vi "quickStack.vi"(2 "stackFname":path=path "C:/Users/sims01/Desktop/dataAcq/data.dcimg", 3 "noFrames":i32, 4 "sCMOShandle":u32, 5 "imgAcqDelay":u32) -> (0 "stackComplete":bool, 1 "timeTaken":u32)   [LabVIEW 2015]
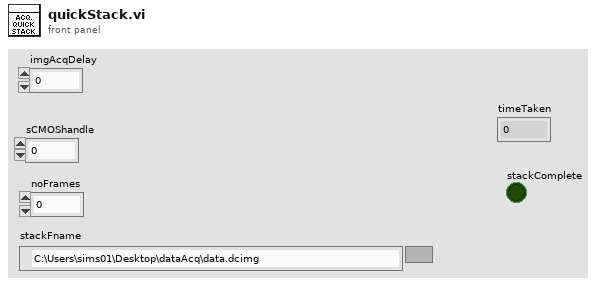
[diagram p1: front panel]
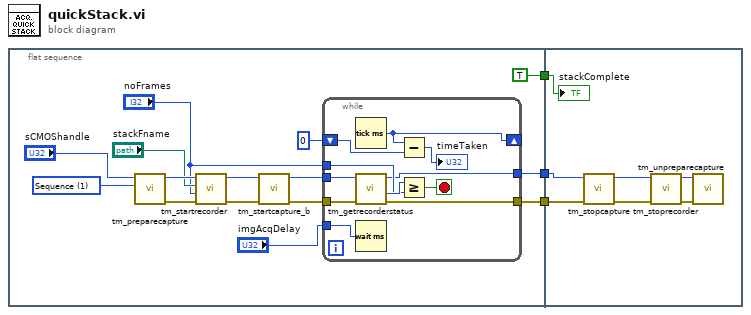
[diagram p0: block diagram]
diagram:
  n1 = flat-sequence {
    tunnel: [TRUE] -> w3
    tunnel: [w5] -> w2
    tunnel: [w6] -> w1
    tunnel: w3 -> [w32]
    tunnel: w2 -> [w31]
    tunnel: w1 -> [w30]
    frame #0 {
      w17 = 1 items=["Snap", "Sequence"] ("Capture mode")
      n2 = call <userlib>:"tm_preparecapture.vi"("Capture mode"=w17, "Handle in"="sCMOShandle") -> ("error out"=w15:errorcluster, "Handle out"=w18:u32)  [unwired: 6 in, 2 out]
      n3 = call <userlib>:"tm_startrecorder.vi"("error in (no error)"=w15, "frames"="noFrames", "File"="stackFname", "Handle in"=w18) -> ("error out"=w14:errorcluster, "Handle out"=w16:u32)  [unwired: 6 in]
      n4 = call <userlib>:"tm_startcapture_b.vi"("error in (no error)"=w14, "Handle in"=w16) -> ("error out"=w7:errorcluster, "Handle out"=w8:u32)  [unwired: 8 in]
      n5 = while {
        tunnel: "noFrames" -> [w27]
        tunnel: w7 -> [w26]
        tunnel: [w25] -> w5
        tunnel: [w24] -> w6
        tunnel: w8 -> [w23]
        tunnel: "imgAcqDelay" -> [w22]
        shift-right: [w19] -> _
        shift-left: u32 0 ("y") -> [w20]
        stop <- w28 stop-if-true
        n6 = Tick Count (ms)() -> (millisecond timer value=w19:u32)
        n7 = call <userlib>:"tm_getrecorderstatus.vi"("error in (no error)"=w26, "Handle"=w23) -> ("error out"=w25:errorcluster, "Count"=w29:i32, "Handle"=w24:u32)  [unwired: 6 in, 1 out]
        n8 = Wait (ms)(milliseconds to wait=w22) -> ()  [unwired: 1 out]
        n9 = Subtract(x=w19, y=w20) -> (x-y=→"timeTaken":u32)
        n10 = Greater Or Equal?(x=w29, y=w27) -> (x >= y?=w28:bool)
      }
    }
    frame #1 {
      n11 = call <userlib>:"tm_stopcapture.vi"("error in (no error)"=w31, "Handle in"=w30) -> ("error out"=w34:errorcluster, "Handle out"=w33:u32)  [unwired: 8 in]
      n12 = call <userlib>:"tm_stoprecorder.vi"("error in (no error)"=w34, "Handle in"=w33) -> ("error out"=w35:errorcluster, "Handle out"=w36:u32)  [unwired: 8 in]
      n13 = call <userlib>:"tm_unpreparecapture.vi"("error in (no error)"=w35, "Handle in"=w36) -> ()  [unwired: 8 in, 2 out]
      "stackComplete" <- w32
    }
  }
